vi "Charger_Append Shutdown Status.vi"(5 "Status Refnum":T1, 6 "error in":errorcluster, 8 "Base Station Idle":bool) -> (0 "error out":errorcluster {"code" format="%.0x"})   [LabVIEW 2020]
doc: "This function appends an \"IPG Shutdown successfully.\" message to the IPG Status cluster status field, if the \"idle\" flag is TRUE and the error status is clear."
uses:
  Charger_Status Refnum.ctl
  Drivers/Charger Test Set/Charger_Input Control.ctl
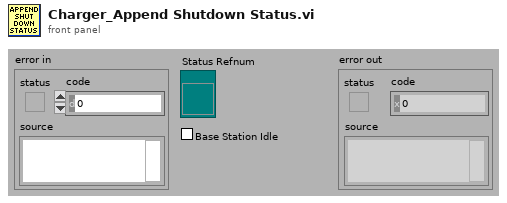
[diagram p1: front panel]
types:
  T1 = typedef "Charger_Status Refnum.ctl" = refnum<vi>
  T2 = typedef "Charger_Input Control.ctl" = cluster{"address":refnum<visa-resource-name>, "position":i32, "setpoint":dbl}
  T3 = cluster{"MICS ID":u32, "VBAT":dbl, "ChargingState":string, "VBAT Slide":dbl, "Status":string, "TemperatureLevel":dbl, "IPG_ReceivedLevel":dbl, "VBAT Target":dbl, "Charger Setpoint":dbl, "Index":i32, "Ready":bool, "Charger Inputs":T2, "MICS Inputs":cluster{"address":refnum<visa-resource-name>, "chan":u16, "ID":u32}}
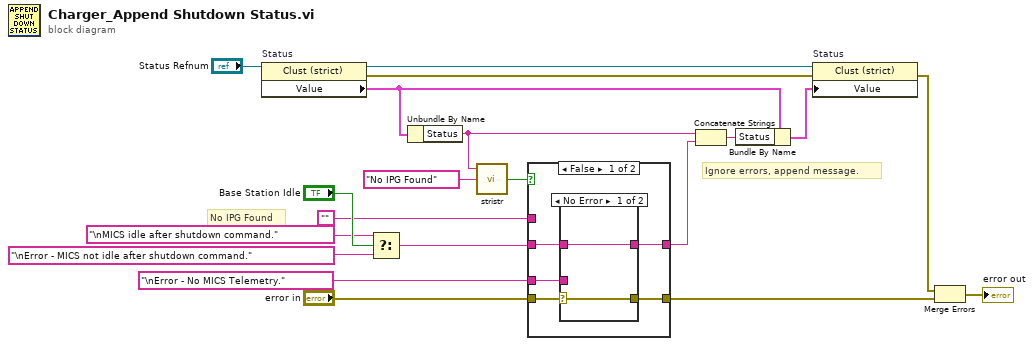
[diagram p0: block diagram]
diagram:
  # "No IPG Found"
  # "Ignore errors, append message."
  n1 = property on="Status" class="Clust (strict)"(reference="Status Refnum") -> (reference out=w18:T1, error out=w19:errorcluster, "Value"=w16:T3)  [unwired: 1 in]
  n2 = Select(t="\nMICS idle after shutdown command." ("status message"), s="Base Station Idle", f="\nError - MICS not idle after shutdown command." ("status message")) -> (s? t:f=w7:string)
  n3 = Unbundle By Name(w16) -> ("Status"=w9:string)
  n4 = call "stristr.vi"("Substring"="No IPG Found" ("regular expression"), "Input String"=w9) -> ("found"=w5:bool)  [unwired: 1 in, 2 out]
  n5 = case shown="False" w5 {
    tunnel: w7 -> [w24 _]
    tunnel: [w23 w31] -> w6
    tunnel: "error in" -> [w25 w30]
    tunnel: "\nError - No MICS Telemetry." ("status message") -> [w22 _]
    tunnel: "" ("status message") -> [_ w31]
    tunnel: [w21 w30] -> w1
    frame False {
      n6 = case shown="No Error" w25 {
        selector: w25 -> [w26 w28]
        tunnel: [w27 w29] -> w23
        tunnel: w24 -> [w27 _]
        tunnel: w22 -> [_ w29]
        tunnel: [w26 w28] -> w21
        frame No Error {
        }
        frame Error {
        }
      }
    }
    frame True {
    }
  }
  n7 = Concatenate Strings(w9, w6) -> (w14:string)
  n8 = Bundle By Name(cluster=w16, "Status"=w14) -> (w15:T3)
  n9 = property on="Status" class="Clust (strict)"(reference=w18, error in=w19, "Value"=w15) -> (error out=w13:errorcluster)  [unwired: 1 out]
  n10 = Merge Errors(w13, w1) -> (→"error out":errorcluster)
